vi "thermo_clusterize_single_channel.vi"(1 "pres":dbl[](array[numeric]), 2 "RH":dbl[](array[numeric]), 3 "temp":dbl[](array[numeric])) -> (0 "thermo channel out":T1[](array[typedef]))   [LabVIEW 2020]
uses:
  thermo_read.ctl
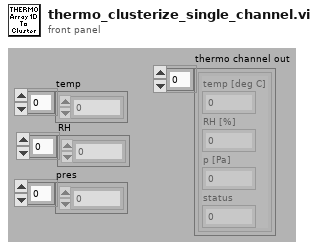
[diagram p1: front panel]
types:
  T1 = typedef "thermo_read.ctl" = cluster{"temp [deg C]":dbl, "RH [%]":dbl, "p [Pa]":dbl, "status":i32}
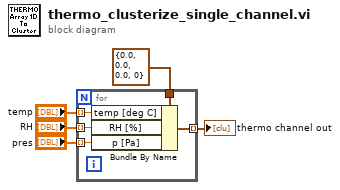
[diagram p0: block diagram]
diagram:
  n1 = for {
    tunnel: "temp" -> [w10] mode=indexing
    tunnel: "RH" -> [w9] mode=indexing
    tunnel: "pres" -> [w8] mode=indexing
    tunnel: T1 {"temp [deg C]"=0.0, "RH [%]"=0.0, "p [Pa]"=0.0, "status"=0} ("thermo") -> [w7]
    tunnel: [w6] -> w1 mode=indexing
    n2 = Bundle By Name(cluster=w7, "temp [deg C]"=w10, "RH [%]"=w9, "p [Pa]"=w8) -> (w6:T1)
  }
  "thermo channel out" <- w1
